vi "Parse Query.vi"(8 "error in (no error)":errorcluster, 11 "URI in":refnum<class "URI.lvclass">) -> (0 "error out":errorcluster, 3 "URI out":refnum<class "URI.lvclass">)   [LabVIEW 2020, in "IO.lvlib" / "URI.lvclass"]
uses:
  URI.lvclass
  URI.lvclass/URI.ctl
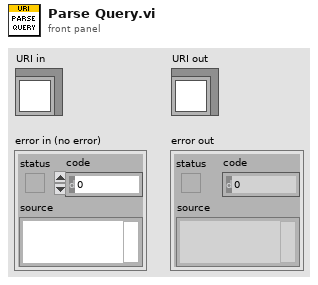
[diagram p1: front panel]
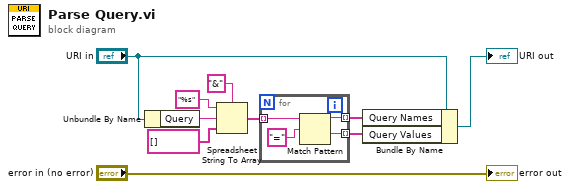
[diagram p0: block diagram]
diagram:
  n1 = Unbundle By Name("URI in") -> ("Query"=w9:string)
  n2 = Spreadsheet String To Array(delimiter (Tab)="&", format string="%s", spreadsheet string=w9, array type (2D Dbl)=string[] []) -> (array=w5:string[])
  n3 = for {
    tunnel: w5 -> [w14] mode=indexing
    tunnel: [w12] -> w1 mode=indexing
    tunnel: [w11] -> w2 mode=indexing
    n4 = Match Pattern(string=w14, regular expression="=") -> (before substring=w11:string, after substring=w12:string)  [unwired: 1 in, 2 out]
  }
  n5 = Bundle By Name(cluster="URI in", "Query Names"=w2, "Query Values"=w1) -> (→"URI out":refnum<class "URI.lvclass">)
  "error out" <- "error in (no error)"
